vi "Get Target IP Address.vi"(8 "error in":errorcluster, 11 "Item Ref in":T1 format="%.0x") -> (0 "error out":errorcluster, 2 "Target IP Address":string, 3 "Item Ref out":T1 format="%.0x")   [LabVIEW 2026, in "SEECD System Explorer.lvlib"]
uses:
  SEECD System Explorer.lvlib
  <vilib>/NI VeriStand/Custom Device Tools/Custom Device Utility Library/Custom Device Utility Library.lvlib
  <vilib>/NI VeriStand/Custom Device Offline API/Custom Device Offline API.lvlib
  NationalInstruments.VeriStand.SystemDefinitionAPI
  C:/Users/Administrator/Desktop/Jatin/All DNC DLLs/NationalInstruments.VeriStand.SystemDefinitionAPI.dll
  Jatin/All DNC DLLs/NationalInstruments.VeriStand.SystemDefinitionAPI.dll
  <vilib>/NI VeriStand/Custom Device API/Custom Device Item Ref.ctl
  <vilib>/NI VeriStand/Custom Device API/Custom Device API.lvlib
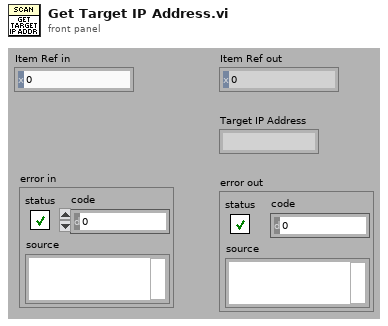
[diagram p1: front panel]
types:
  T1 = typedef "Custom Device API.lvlib/Custom Device Item Ref.ctl" = u64
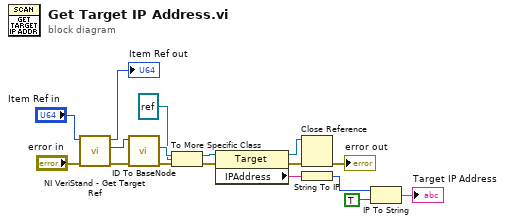
[diagram p0: block diagram]
diagram:
  n1 = call <vilib>:"NI VeriStand - Get Target Ref.vi"("error in"="error in", "Item Ref in"="Item Ref in") -> ("error out"=w1:errorcluster, "Target Ref"=w9:T1, "Item Ref out"=→"Item Ref out":T1)  [unwired: 6 in, 1 out]
  n2 = call <vilib>:"ID To BaseNode.vi"("error in (no error)"=w1, "ID in"=w9) -> ("error out"=w4:errorcluster, "BaseNode"=w3:refnum<k24>)  [unwired: 7 in, 1 out]
  n3 = To More Specific Class(target class=refnum<k39> refnum, reference=w3, error in=w4) -> (specific class reference=w5:refnum<k39>, error out=w6:errorcluster)
  n4 = property class="Target"(reference=w5, error in=w6) -> (reference out=w7:refnum<k39>, error out=w8:errorcluster, "IPAddress"=w12:string)
  n5 = Close Reference(reference=w7, error in (no error)=w8) -> (error out=→"error out":errorcluster)
  n6 = String To IP(1:w12) -> (0:w10:u32)
  n7 = IP To String(1:TRUE ("dot notation? (F)"), 2:w10) -> (0:→"Target IP Address":string)
